vi "Unified Actor Lifetime.vi"(7 "Actor in":refnum<class "Actor.lvclass">, 10 "Unified Actor Lifetime":T1) -> (5 "Actor out":refnum<class "Actor.lvclass">)   [LabVIEW 2025, in "Base Actor.lvlib"]
uses:
  Base Actor/Base Actor.lvlib
  Actor/Actor.lvclass
  Unified Actor Lifetime.ctl
  jettl.lvlib
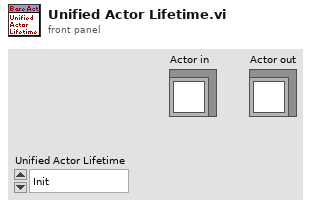
[diagram p1: front panel]
types:
  T1 = typedef "jettl.lvlib/Unified Actor Lifetime.ctl" = enum16{"Init", "Spawn", "Setup", "Teardown Before Running", "Running", "Stop Called", "Stopping With Children", "Stopping Without Children", "Teardown After Running", "Stopped"}
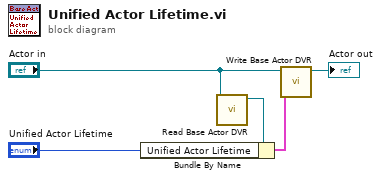
[diagram p0: block diagram]
diagram:
  n1 = call-dynamic "Read Base Actor DVR.vi"("Actor in"="Actor in") -> ("Base Actor DVR"=w3:refnum<data-value>)  [unwired: 10 in]
  n2 = Bundle By Name(cluster=w3, "Unified Actor Lifetime"="Unified Actor Lifetime") -> (w2:cluster{})
  n3 = call-dynamic "Write Base Actor DVR.vi"("Base Actor DVR"=w2, "Actor in"="Actor in") -> ("Actor out"=→"Actor out":refnum<class "Actor.lvclass">)  [unwired: 9 in]
